vi "m2Testing.vi"() -> ()   [LabVIEW 2015]
uses:
  Common_RT_ILC/DataTypes/ILCTelemetry.ctl
  Common_RT_ILC/DataTypes/ILCResponses.ctl
  Common_RT_Modbus/DataTypes/ExceptionCodes.ctl
  Common_RT_HPILC/DataTypes/HPResponses.ctl
  Common_RT_HPILC/DataTypes/HPTelemetry.ctl
  Common_RT_HealthAndStatus/RTHealthAndStatus/RTHealthAndStatus.lvclass
  MyHealthAndStatusReadFIFO/MyHealthAndStatusReadFIFO.lvclass
  MyHealthAndStatusWriteFIFO/MyHealthAndStatusWriteFIFO.lvclass
  Common_RT_Modbus/Modbus/Modbus.lvclass
  ModbusPort1ReadFIFO/ModbusPort1ReadFIFO.lvclass
  ModbusPort1WriteFIFO/ModbusPort1WriteFIFO.lvclass
  SoftwareControlledTrigger/SoftwareControlledTrigger.lvclass
  Common_RT_HPILC/HPILCFactory/HPILCFactory.lvclass
  Common_RT_HPILC/DataTypes/HPSettings.ctl
  Common_RT_ILC/DataTypes/ILCSettings.ctl
  SoftwareControlledTrigger/SoftwareControlledTrigger.lvclass/SoftwareControlledTrigger.ctl
  ModbusPort1WriteFIFO/ModbusPort1WriteFIFO.lvclass/ModbusPort1WriteFIFO.ctl
  ModbusPort1ReadFIFO/ModbusPort1ReadFIFO.lvclass/ModbusPort1ReadFIFO.ctl
  Common_RT_Modbus/Modbus/Modbus.lvclass/Modbus.ctl
  MyHealthAndStatusWriteFIFO/MyHealthAndStatusWriteFIFO.lvclass/MyHealthAndStatusWriteFIFO.ctl
  MyHealthAndStatusReadFIFO/MyHealthAndStatusReadFIFO.lvclass/MyHealthAndStatusReadFIFO.ctl
  Common_RT_HealthAndStatus/RTHealthAndStatus/RTHealthAndStatus.lvclass/RTHealthAndStatus.ctl
  Common_RT_ILC/ILC/ILC.lvclass/ILC.ctl
  Common_RT_Modbus/DynamicFrameParser/DynamicFrameParser.lvclass
  Common_RT_HPILC/HPILC/HPILC.lvclass/HPILC.ctl
  <vilib>/FPGAPlugInAG/cRIO-9038/niLvFpga_Open_cRIO-9038.vi
  <vilib>/rvi/interface/common/dynamic/niFpgaDynamicAddResources.vi
  <vilib>/FPGAPlugInAG/Dynamic/niLvFpga_Abort_Dynamic.vi
  <vilib>/FPGAPlugInAG/Dynamic/niLvFpga_Reset_Dynamic.vi
  <vilib>/FPGAPlugInAG/Dynamic/niLvFpga_Run_Dynamic.vi
  <vilib>/FPGAPlugInAG/Dynamic/niLvFpga_Close_Dynamic.vi
  <vilib>/rvi/interface/nirviOpenFPGA/nirviOpenFPGA.xnode
  FPGA Bitfiles/Modbus-4Port.lvbitx
  FPGA/main.vi
  <vilib>/rvi/interface/nirviMethod/nirviMethod.xnode
  <vilib>/rvi/interface/nirviCloseFPGA/nirviCloseFPGA.xnode
  Common_RT_HPILC/HPILC/HPILC.lvclass
  Common_RT_ILC/RTILC.lvlib
  Common_RT_ILC/ILC/ILC.lvclass
  Common_RT_HPILC/RTHPILC.lvlib
  Common_RT_Modbus/RTModbus.lvlib
panel:
  out "Array":bool[](array[boolean])
  out "HPTelemetry":T1
  out "HPResponses":T2
  in  "Boolean":bool
  out "ILCResponses":T4
  out "ILCTelemetry":T5
  out "Port 1 Status Bits":u64 format="%016b"
  out "error out":errorcluster
  out "Port 1 Frames Received":i64
  out "Port 1 Bytes Received":i64
  out "Port 1 Frames Transmitted":i64
  out "Port 1 Bytes Transmitted":i64
  # "Port 1 = Modbus"
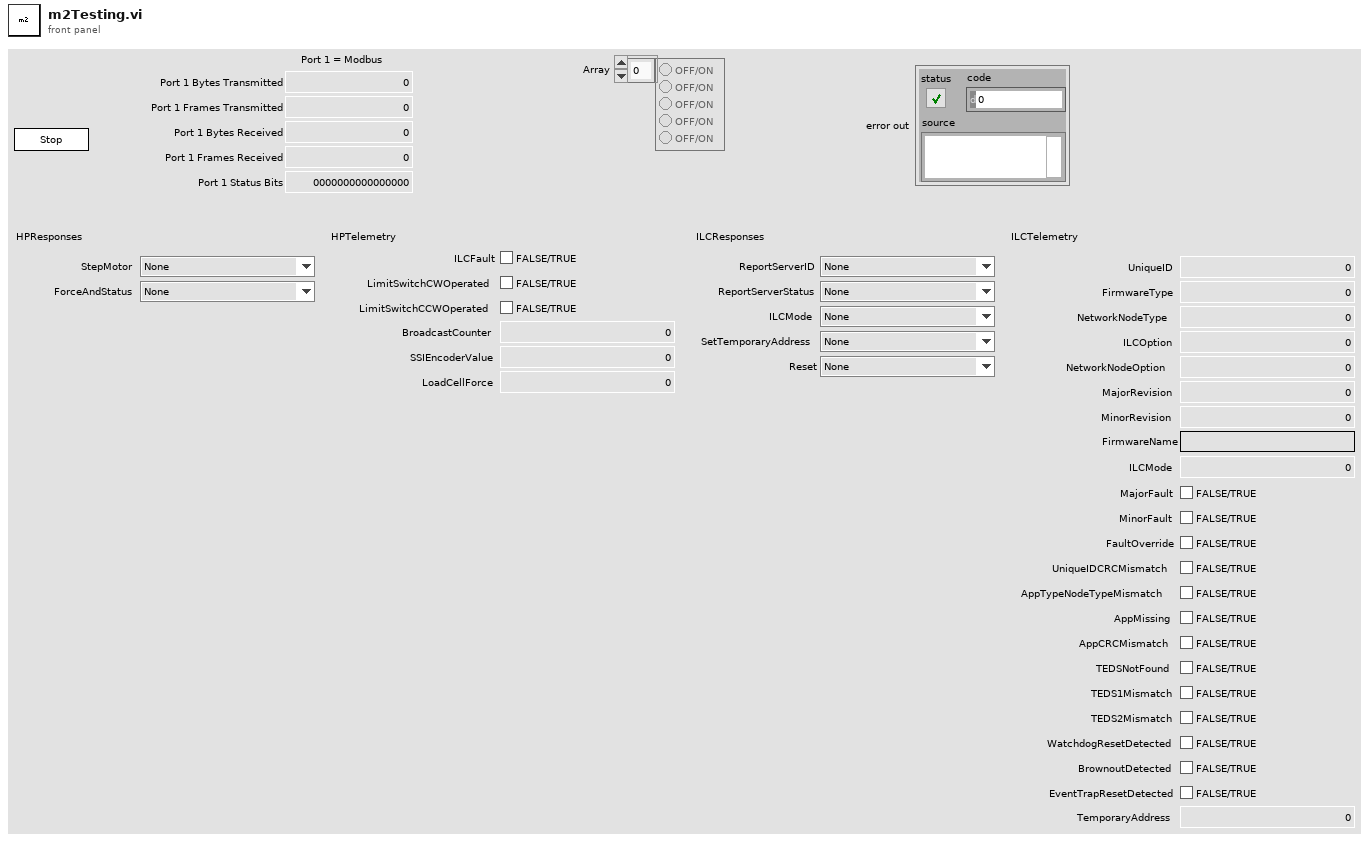
[diagram p1: front panel]
types:
  T1 = typedef "RTHPILC.lvlib/HPTelemetry.ctl" = cluster{"ILCFault":bool, "LimitSwitchCWOperated":bool, "LimitSwitchCCWOperated":bool, "BroadcastCounter":u8, "SSIEncoderValue":i32, "LoadCellForce":sgl}
  T2 = typedef "RTHPILC.lvlib/HPResponses.ctl" = cluster{"StepMotor":T3, "ForceAndStatus":T3}
  T3 = typedef "RTModbus.lvlib/ExceptionCodes.ctl" = enum16{"None", "IllegalFunction", "IllegalDataAddress", "IllegalDataValue", "SlaveDeviceFailure", "Acknowledge", "SlaveDeviceBusy", "NegativeAcknowledge", "MemoryParityError", "GatewayPathUnavailable", "GatewayTargetDeviceFailedToRespond"}
  T4 = typedef "RTILC.lvlib/ILCResponses.ctl" = cluster{"ReportServerID":T3, "ReportServerStatus":T3, "ILCMode":T3, "SetTemporaryAddress":T3, "Reset":T3}
  T5 = typedef "RTILC.lvlib/ILCTelemetry.ctl" = cluster{"UniqueID":u64, "FirmwareType":u8, "NetworkNodeType":u8, "ILCOption":u8, "NetworkNodeOption":u8, "MajorRevision":u8, "MinorRevision":u8, "FirmwareName":string, "ILCMode":u16, "MajorFault":bool, "MinorFault":bool, "FaultOverride":bool, "UniqueIDCRCMismatch":bool, "AppTypeNodeTypeMismatch":bool, "AppMissing":bool, "AppCRCMismatch":bool, "TEDSNotFound":bool, "TEDS1Mismatch":bool, "TEDS2Mismatch":bool, "WatchdogResetDetected":bool, "BrownoutDetected":bool, "EventTrapResetDetected":bool, "TemporaryAddress":u8}
  T6 = typedef "RTHPILC.lvlib/HPSettings.ctl" = cluster{"ILCSettings":T7, "ID":i16, "ReferencePosition":u32}
  T7 = typedef "RTILC.lvlib/ILCSettings.ctl" = cluster{"Subnet":u8, "Address":u8}
  T8 = typedef "RTILC.lvlib/ILCData.ctl" = cluster{"Constants":T9, "Command":T10, "Telemetry":T5, "Responses":T4}
  T9 = typedef "RTILC.lvlib/ILCConstants.ctl" = cluster{"Subnet":u8, "Address":u8}
  T10 = typedef "RTILC.lvlib/ILCCommand.ctl" = cluster{"ILCMode":u16, "TemporaryAddress":u8}
  T11 = typedef "RTModbus.lvlib/Frame.ctl" = cluster{"Data":u8[], "WaitForTrigger":bool, "WaitForRx":u16, "TriggerIRQ":bool}
  T12 = typedef "RTHPILC.lvlib/HPData.ctl" = cluster{"HPConstants":T13, "HPCommand":T14, "HPTelemetry":T1, "HPResponses":T2}
  T13 = typedef "RTHPILC.lvlib/HPConstants.ctl" = cluster{"ID":i16, "ReferencePosition":u32}
  T14 = typedef "RTHPILC.lvlib/HPCommand.ctl" = cluster{"Steps":i8}
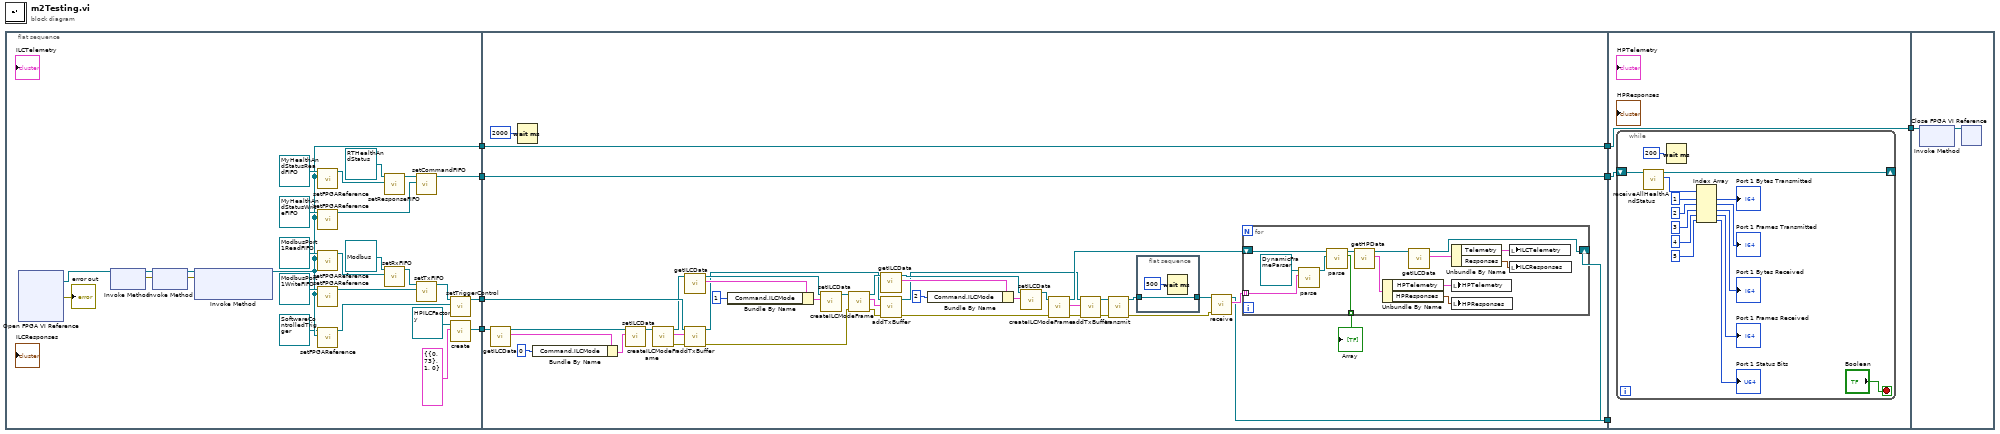
[diagram p0: block diagram]
diagram:
  n1 = flat-sequence {
    tunnel: [w17] -> w9
    tunnel: [w14] -> w6
    tunnel: [w32] -> w5
    tunnel: [w10] -> w3
    tunnel: w9 -> [w78]
    tunnel: [w78] -> w8
    tunnel: w6 -> [w45]
    tunnel: w5 -> [w76]
    tunnel: [w76] -> w4
    tunnel: w3 -> [w46]
    tunnel: [w38] -> w2
    tunnel: [w41] -> w1
    tunnel: w8 -> [w95]
    tunnel: [w95] -> w7
    tunnel: w4 -> [w96]
    tunnel: w2 -> [_]
    tunnel: w1 -> [_]
    tunnel: w7 -> [w112]
    frame #0 {
      n2 = xnode "Open FPGA VI Reference"() -> ("FPGA VI Reference Out"=w19:refnum<k20>, "error out"=→"error out":errorcluster)  [unwired: 2 in]
      n3 = xnode "Invoke Method"("FPGA VI Reference In"=w19) -> ("FPGA VI Reference Out"=w36:refnum<k20>, "error out"=w21:errorcluster)  [unwired: 1 in]
      n4 = xnode "Invoke Method"("FPGA VI Reference In"=w36, "error in"=w21) -> ("FPGA VI Reference Out"=w35:refnum<k20>, "error out"=w20:errorcluster)
      n5 = xnode "Invoke Method"("FPGA VI Reference In"=w35, "error in"=w20) -> ("FPGA VI Reference Out"=w17:refnum<k20>)  [unwired: 1 in, 1 out]
      n6 = call "setFPGAReference.vi"("FPGAReference"=w17, "MyHealthAndStatusReadFIFO in"=refnum<class "MyHealthAndStatusReadFIFO.lvclass"> refnum ("MyHealthAndStatusReadFIFO.lvclass")) -> ("MyHealthAndStatusReadFIFO out"=w28:refnum<class "MyHealthAndStatusReadFIFO.lvclass">)  [unwired: 9 in]
      n7 = call "setFPGAReference.vi"("FPGAReference"=w17, "MyHealthAndStatusWriteFIFO in"=refnum<class "MyHealthAndStatusWriteFIFO.lvclass"> refnum ("MyHealthAndStatusWriteFIFO.lvclass")) -> ("MyHealthAndStatusWriteFIFO out"=w26:refnum<class "MyHealthAndStatusWriteFIFO.lvclass">)  [unwired: 9 in]
      n8 = call "setFPGAReference.vi"("FPGAReference"=w17, "ModbusPort1ReadFIFO in"=refnum<class "ModbusPort1ReadFIFO.lvclass"> refnum ("ModbusPort1ReadFIFO.lvclass")) -> ("ModbusPort1ReadFIFO out"=w24:refnum<class "ModbusPort1ReadFIFO.lvclass">)  [unwired: 9 in]
      n9 = call "setFPGAReference.vi"("FPGAReference"=w17, "ModbusPort1WriteFIFO in"=refnum<class "ModbusPort1WriteFIFO.lvclass"> refnum ("ModbusPort1WriteFIFO.lvclass")) -> ("ModbusPort1WriteFIFO out"=w22:refnum<class "ModbusPort1WriteFIFO.lvclass">)  [unwired: 9 in]
      n10 = call "setFPGAReference.vi"("FPGAReference"=w17, "SoftwareControlledTrigger in"=refnum<class "SoftwareControlledTrigger.lvclass"> refnum ("SoftwareControlledTrigger.lvclass")) -> ("SoftwareControlledTrigger out"=w13:refnum<class "SoftwareControlledTrigger.lvclass">)  [unwired: 9 in]
      n11 = call "setResponseFIFO.vi"("ReadU32FIFO"=w28, "RTHealthAndStatus in"=refnum<class "RTHealthAndStatus.lvclass"> refnum ("RTHealthAndStatus.lvlib:RTHealthAndStatus.lvclass")) -> ("RTHealthAndStatus out"=w33:refnum<class "RTHealthAndStatus.lvclass">)  [unwired: 9 in]
      n12 = call "setRxFIFO.vi"("ReadU16FIFO"=w24, "Modbus in"=refnum<class "Modbus.lvclass"> refnum ("RTModbus.lvlib:Modbus.lvclass")) -> ("Modbus out"=w30:refnum<class "Modbus.lvclass">)  [unwired: 9 in]
      n13 = call "setCommandFIFO.vi"("WriteU64FIFO"=w26, "RTHealthAndStatus in"=w33) -> ("RTHealthAndStatus out"=w32:refnum<class "RTHealthAndStatus.lvclass">)  [unwired: 9 in]
      n14 = call "setTxFIFO.vi"("WriteU16FIFO"=w22, "Modbus in"=w30) -> ("Modbus out"=w15:refnum<class "Modbus.lvclass">)  [unwired: 9 in]
      n15 = call "setTriggerControl.vi"("TriggerControl"=w13, "Modbus in"=w15) -> ("Modbus out"=w14:refnum<class "Modbus.lvclass">)  [unwired: 9 in]
      n16 = call "create.vi"("HPSettings"=T6 {"ILCSettings"={"Subnet"=0, "Address"=73}, "ID"=1, "ReferencePosition"=0}, "HardPointActuatorFactory in"=refnum<class "HPILCFactory.lvclass"> refnum ("RTHPILC.lvlib:HPILCFactory.lvclass")) -> ("HardPointActuator"=w10:refnum<class "HPILC.lvclass">)  [unwired: 7 in, 2 out]
    }
    frame #1 {
      n17 = call "getILCData.vi"("ILC in"=w46) -> ("ILCData"=w47:T8, "ILC out"=w51:refnum<class "HPILC.lvclass">)  [unwired: 9 in]
      n18 = Wait (ms)(milliseconds to wait=u32 2000) -> ()  [unwired: 1 out]
      n19 = Bundle By Name(cluster=w47, "Command.ILCMode"=u16 0) -> (w49:T8)
      n20 = call "setILCData.vi"("ILCData"=w49, "ILC in"=w51) -> ("ILC out"=w50:refnum<class "HPILC.lvclass">)  [unwired: 9 in]
      n21 = call "createILCModeFrame.vi"("ILC in"=w50) -> ("error out"=w53:errorcluster, "Frame"=w52:T11, "ILC out"=w42:refnum<class "HPILC.lvclass">)  [unwired: 8 in]
      n22 = call "getILCData.vi"("ILC in"=w42) -> ("ILCData"=w75:T8, "ILC out"=w65:refnum<class "HPILC.lvclass">)  [unwired: 9 in]
      n23 = call "addTxBuffer.vi"("error in (no error)"=w53, "Frame"=w52, "Modbus in"=w45) -> ("error out"=w39:errorcluster, "Modbus out"=w40:refnum<class "Modbus.lvclass">)  [unwired: 7 in]
      n24 = Bundle By Name(cluster=w75, "Command.ILCMode"=u16 1) -> (w73:T8)
      n25 = call "setILCData.vi"("ILCData"=w73, "ILC in"=w65) -> ("ILC out"=w66:refnum<class "HPILC.lvclass">)  [unwired: 9 in]
      n26 = call "createILCModeFrame.vi"("error in (no error)"=w39, "ILC in"=w66) -> ("error out"=w62:errorcluster, "Frame"=w64:T11, "ILC out"=w67:refnum<class "HPILC.lvclass">)  [unwired: 7 in]
      n27 = call "getILCData.vi"("ILC in"=w67) -> ("ILCData"=w72:T8, "ILC out"=w69:refnum<class "HPILC.lvclass">)  [unwired: 9 in]
      n28 = call "addTxBuffer.vi"("error in (no error)"=w62, "Frame"=w64, "Modbus in"=w40) -> ("error out"=w43:errorcluster, "Modbus out"=w44:refnum<class "Modbus.lvclass">)  [unwired: 7 in]
      n29 = Bundle By Name(cluster=w72, "Command.ILCMode"=u16 2) -> (w70:T8)
      n30 = call "setILCData.vi"("ILCData"=w70, "ILC in"=w69) -> ("ILC out"=w68:refnum<class "HPILC.lvclass">)  [unwired: 9 in]
      n31 = call "createILCModeFrame.vi"("error in (no error)"=w43, "ILC in"=w68) -> ("error out"=w61:errorcluster, "Frame"=w63:T11, "ILC out"=w54:refnum<class "HPILC.lvclass">)  [unwired: 7 in]
      n32 = call "addTxBuffer.vi"("error in (no error)"=w61, "Frame"=w63, "Modbus in"=w44) -> ("error out"=w59:errorcluster, "Modbus out"=w60:refnum<class "Modbus.lvclass">)  [unwired: 7 in]
      n33 = call "transmit.vi"("error in (no error)"=w59, "Modbus in"=w60) -> ("error out"=w56:errorcluster, "Modbus out"=w58:refnum<class "Modbus.lvclass">)  [unwired: 8 in]
      n34 = flat-sequence {
        tunnel: [w93] -> w57
        tunnel: w58 -> [w93]
        frame #0 {
          n35 = Wait (ms)(milliseconds to wait=u32 500) -> ()  [unwired: 1 out]
        }
      }
      n36 = call "receive.vi"("error in (no error)"=w56, "Modbus in"=w57) -> ("Data"=w55:T11[], "Modbus out"=w38:refnum<class "Modbus.lvclass">)  [unwired: 7 in, 1 out]
      n37 = for {
        tunnel: w55 -> [w92] mode=indexing
        shift-right: [w81] -> w41
        shift-left: w54 -> [w89]
        tunnel: [w79] -> w37 mode=indexing
        n38 = call "parse.vi"("Frame"=w92, "FrameParser in"=refnum<class "DynamicFrameParser.lvclass"> refnum ("RTModbus.lvlib:DynamicFrameParser.lvclass")) -> ("FrameParser out"=w90:refnum<class "DynamicFrameParser.lvclass">)  [unwired: 8 in, 1 out]
        n39 = call-dynamic "parse.vi"("DynamicFrameParser"=w90, "HPILC in"=w89) -> ("ParseSuccessful"=w79:bool, "HPILC out"=w80:refnum<class "HPILC.lvclass">)  [unwired: 7 in, 1 out]
        n40 = call "getHPData.vi"("HardPointActuator in"=w80) -> ("HPData"=w82:T12, "HardPointActuator out"=w88:refnum<class "HPILC.lvclass">)  [unwired: 9 in]
        n41 = Unbundle By Name(w82) -> ("HPTelemetry"=w83:T1, "HPResponses"=w84:T2)
        n42 = call "getILCData.vi"("ILC in"=w88) -> ("ILCData"=w85:T8, "ILC out"=w81:refnum<class "HPILC.lvclass">)  [unwired: 9 in]
        n43 = Unbundle By Name(w85) -> ("Telemetry"=w86:T5, "Responses"=w87:T4)
        n44 = local write "HPTelemetry"(w83) -> ()
        n45 = local write "HPResponses"(w84) -> ()
        n46 = local write "ILCTelemetry"(w86) -> ()
        n47 = local write "ILCResponses"(w87) -> ()
      }
      "Array" <- w37
    }
    frame #2 {
      n48 = while {
        shift-right: [w109] -> _
        shift-left: w96 -> [w110]
        stop <- "Boolean" stop-if-true
        n49 = call "receiveAllHealthAndStatus.vi"("RTHealthAndStatus in"=w110) -> ("Data"=w104:u32[], "RTHealthAndStatus out"=w109:refnum<class "RTHealthAndStatus.lvclass">)  [unwired: 8 in, 1 out]
        n50 = Wait (ms)(milliseconds to wait=u32 200) -> ()  [unwired: 1 out]
        n51 = Index Array(array=w104, index #1=1 ("index"), index #2=2 ("index"), index #3=3 ("index"), index #4=4 ("index"), index #5=5 ("index")) -> (element #1=→"Port 1 Bytes Transmitted":u32, element #2=→"Port 1 Frames Transmitted":u32, element #3=→"Port 1 Bytes Received":u32, element #4=→"Port 1 Frames Received":u32, element #5=→"Port 1 Status Bits":u32)
      }
    }
    frame #3 {
      n52 = xnode "Invoke Method"("FPGA VI Reference In"=w112) -> ("FPGA VI Reference Out"=w113:refnum<k20>)  [unwired: 1 in, 1 out]
      n53 = xnode "Close FPGA VI Reference"("FPGA VI Reference In"=w113) -> ()  [unwired: 1 in, 1 out]
    }
  }
